vi "Magnet Filter.vi"(1 "Magnet":T1, 3 "seq in":string[][](array[string])=[["0", "", "100"], ["1", "", "1"], ["2", "", "1"], ["3", "", "1"], ["4", "", "1"], ["5", "", "1"], ["6", "", "1"], ["7", "", "1"], ["8", "", "100"]]) -> (0 "seq  out":string[][](array[string]))   [LabVIEW 2020]
uses:
  Ctl/magnet.ctl
panel:
  out "32bit integer":i32
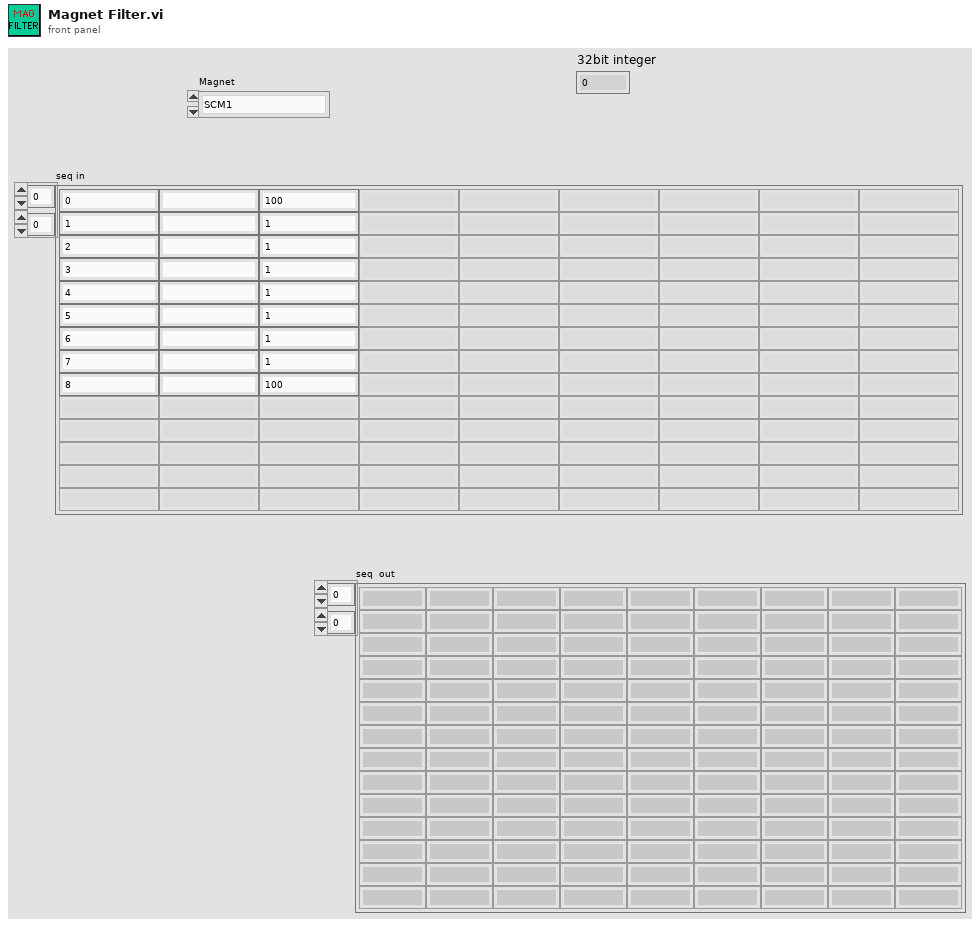
[diagram p1: front panel]
types:
  T1 = typedef "magnet.ctl" = enum16{"SCM1", "SCM2", "SCM3", "SCMX", "Cell8", "Cell9", "Cell12", "Hybrid", "Great Magnet"}
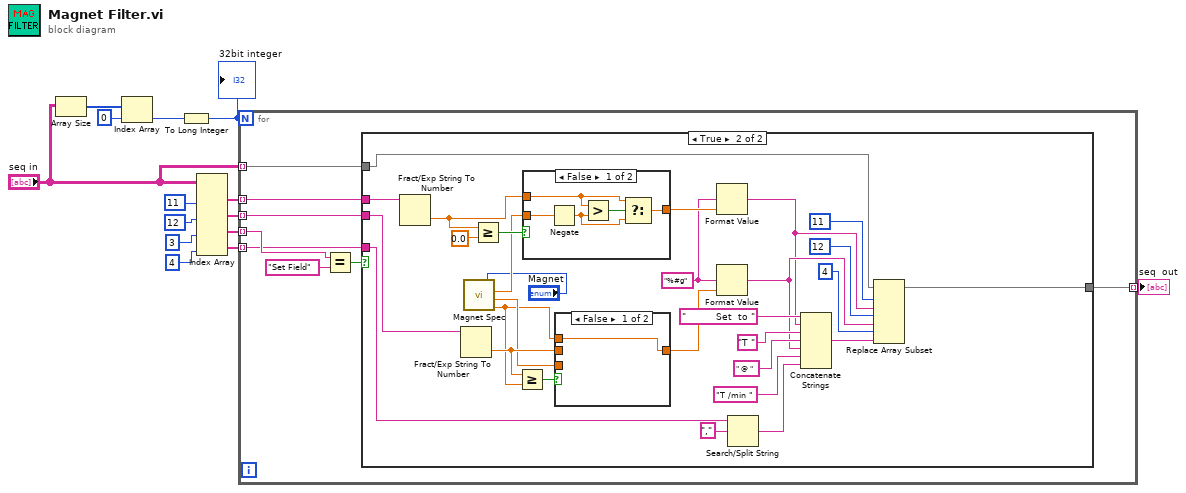
[diagram p0: block diagram]
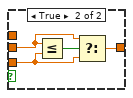
[diagram p3: hidden frame]
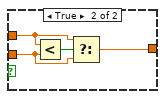
[diagram p4: hidden frame]
diagram:
  n1 = Array Size(array="seq in") -> (size(s)=w3:i32[])
  n2 = Index Array(array=w3, index=0) -> (element=w1:i32)
  n3 = To Long Integer(number=w1) -> (32bit integer=w14:i32)
  "32bit integer" <- w14
  n4 = Index Array(array="seq in", index (col) #1=11 ("disabled index (col)"), index (col) #2=12 ("index (col)"), index (col) #3=3 ("index (col)"), index (col) #4=4 ("index (col)")) -> (element #1=w13:string[], element #2=w10:string[], element #3=w8:string[], element #4=w5:string[])  [unwired: 4 in]
  n5 = for {
    N: w14 -> [_]
    tunnel: w13 -> [w22] mode=indexing
    tunnel: w10 -> [w21] mode=indexing
    tunnel: w8 -> [w19] mode=indexing
    tunnel: "seq in" -> [w17] mode=indexing
    tunnel: [w16] -> w7 mode=indexing
    tunnel: w5 -> [w15] mode=indexing
    n6 = Equal?(x=w19, y="Set Field") -> (x = y?=w18:bool)
    n7 = case shown="True" w18 {
      tunnel: w22 -> [_ w52]
      tunnel: w21 -> [_ w51]
      tunnel: [w23 w40] -> w16
      tunnel: w17 -> [w23 w41]
      tunnel: w15 -> [_ w38]
      frame False {
      }
      frame True {
        w34 = "%#g" ("format string")
        n8 = Fract/Exp String To Number(string=w52) -> (number=w48:dbl)  [unwired: 3 in, 1 out]
        n9 = Fract/Exp String To Number(string=w51) -> (number=w45:dbl)  [unwired: 3 in, 1 out]
        n10 = call "Magnet Spec.vi"("Magnet"="Magnet") -> ("min rate (T/min)"=w25:dbl, "max rate (T/min)"=w44:dbl, "max field (T)"=w47:dbl)  [unwired: 1 in, 4 out]
        n11 = Greater Or Equal?(x=w48, y=0.0) -> (x >= y?=w50:bool)
        n12 = Greater Or Equal?(x=w45, y=w25) -> (x >= y?=w46:bool)
        n13 = case shown="False" w50 {
          tunnel: w48 -> [w60 w65]
          tunnel: w47 -> [w62 w64]
          tunnel: [w58 w63] -> w36
          frame False {
            n14 = Negate(x=w62) -> (-x=w59:dbl)
            n15 = Greater?(x=w60, y=w59) -> (0:w61:bool)
            n16 = Select(t=w60, s=w61, f=w59) -> (s? t:f=w58:dbl)
          }
          frame True {
            n17 = Less?(x=w65, y=w64) -> (x < y?=w66:bool)
            n18 = Select(t=w65, s=w66, f=w64) -> (s? t:f=w63:dbl)
          }
        }
        n19 = case shown="False" w46 {
          tunnel: w45 -> [_ w56]
          tunnel: w44 -> [_ w55]
          tunnel: [w53 w54] -> w35
          tunnel: w25 -> [w53 _]
          frame False {
          }
          frame True {
            n20 = Less Or Equal?(x=w56, y=w55) -> (x <= y?=w57:bool)
            n21 = Select(t=w56, s=w57, f=w55) -> (s? t:f=w54:dbl)
          }
        }
        n22 = Format Value(format string=w34, value (0)=w36) -> (output string=w27:string)  [unwired: 1 in]
        n23 = Format Value(format string=w34, value (0)=w35) -> (output string=w28:string)  [unwired: 1 in]
        n24 = Search/Split String(string=w38, search string/char (-)=",") -> (match + rest of string=w29:string)  [unwired: 1 in, 2 out]
        n25 = Concatenate Strings("          Set  to " ("string"), w27, "T " ("string"), " @ " ("string"), w28, "T /min " ("string"), w29) -> (w26:string)
        n26 = Replace Array Subset(array=w41, new element #1=w27, index #1=11 ("index"), new element #2=w28, index #2=12 ("index"), new element #3=w26, index #3=4 ("index")) -> (w40:string[])
      }
    }
  }
  "seq  out" <- w7
